vi "SDSU_REGS.vi"(0 "refnum":i32, 5 "Command":string, 7 "physical unit":string, 9 "swhitches":string[](array[string]), 11 "error in (no error)":errorcluster, 12 "switch arguments":string[](array[string])) -> (4 "refnum out":i32, 6 "response":string, 15 "error out":errorcluster)   [LabVIEW 2016]
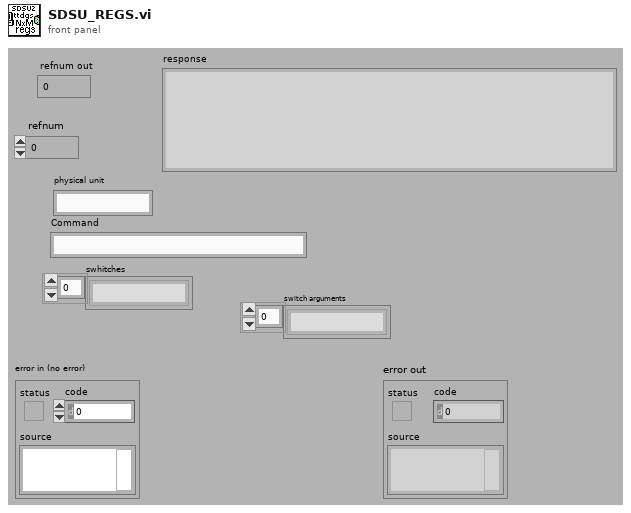
[diagram p1: front panel]
types:
  T1 = enum16{"READ FROM FILE", "GET ALL", "FIND BY NAME", "SET FIELD VALUE", "CLEAN"}
  T2 = typedef "CMN_ContStatus.ctl" = cluster{"Response":string, "power":bool, "shutter":bool, "artifdata":bool, "idlemode":bool, "reset":bool, "gain":u8, "speed":u8, "resetPCI":bool, "autoshutter":bool, "TempSetPoint":i32, "multipleextensions":bool, "displayImage":bool, "coadding":bool, "images being coadded":i32, "Operation Mode":enum16{"normal", "coadd", "fawler"}, "frames to write":cluster{"subs":bool, "reset":bool, "exposed":bool}, "fawler samples":i32, "write auto":bool, "datatype":string, "frames to display":cluster{"subs":bool, "reset":bool, "exposed":bool}, "sur":i32, "autoclear":bool}
  T3 = typedef "SDSU_Register.ctl" = cluster{"Name":string, "address":i16, "width":i16, "comment":string, "Fields":T4[], "value":string}
  T4 = typedef "SDSU_RegField.ctl" = cluster{"name":string, "position":u16, "num_bits":u16, "default":i16, "comment":string, "value":i32}
  T5 = enum16{"Idle", "Exposing", "Paused", "AbortExp", "Reading", "AbortRead", "FinishedReading", "Resetting", "Reducing", "Initializing"}
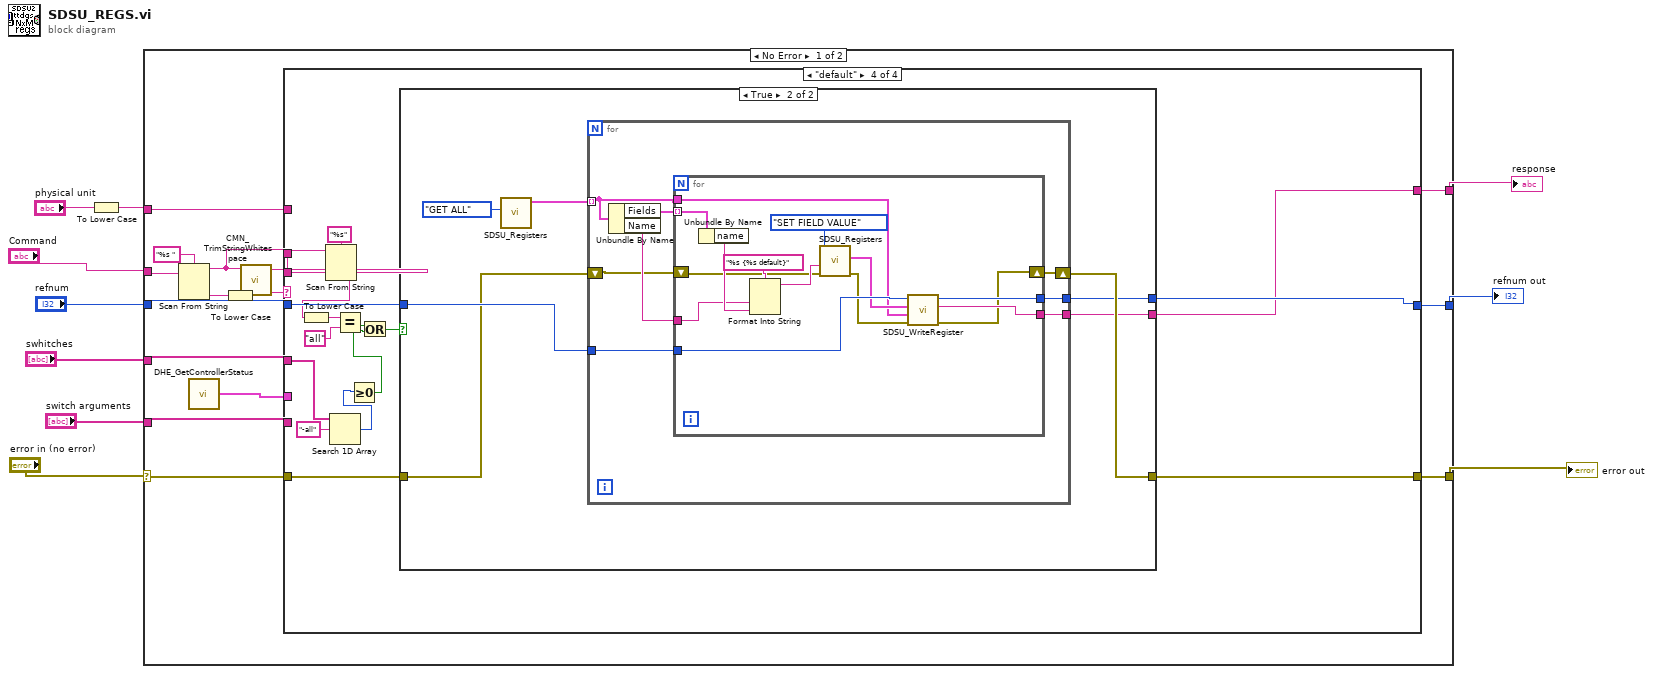
[diagram p0: block diagram]
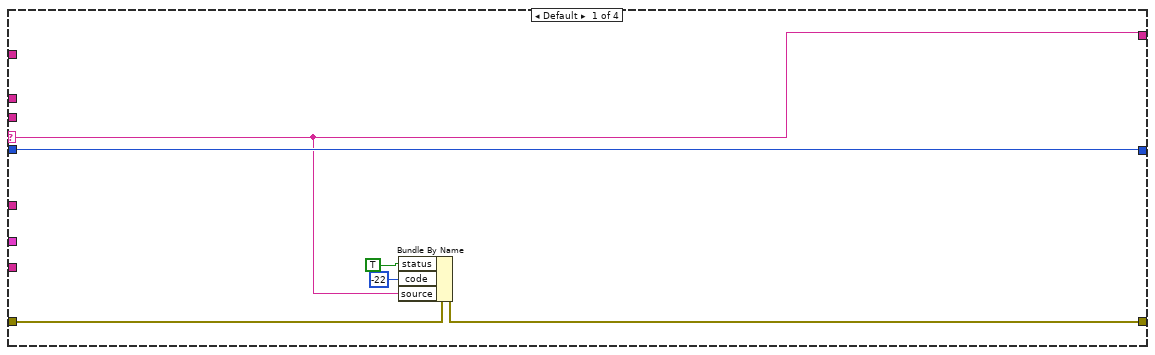
[diagram p2: hidden frame]
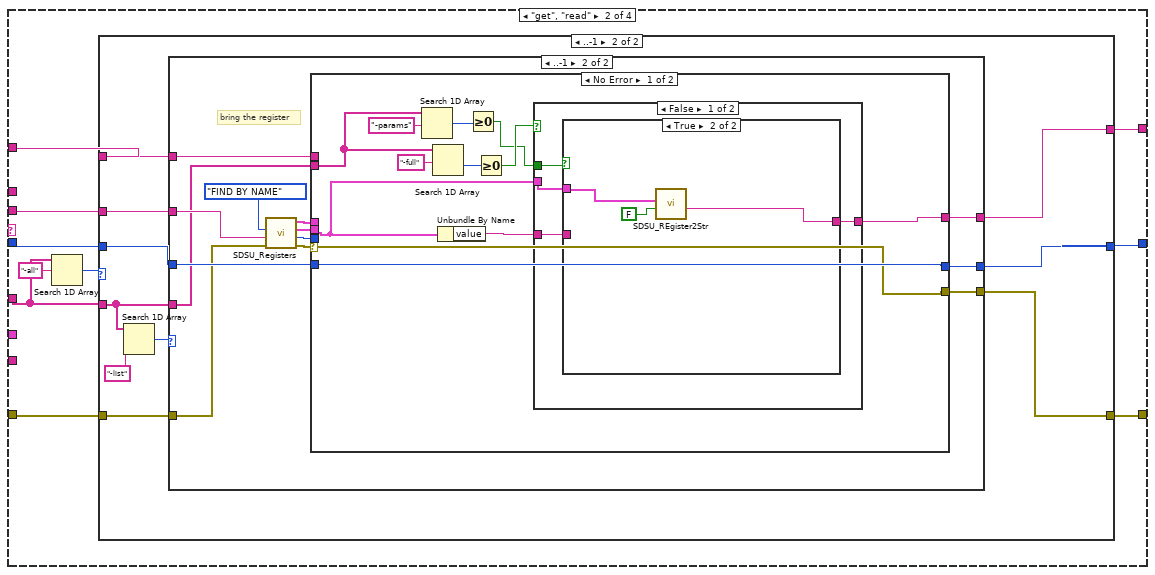
[diagram p3: hidden frame]
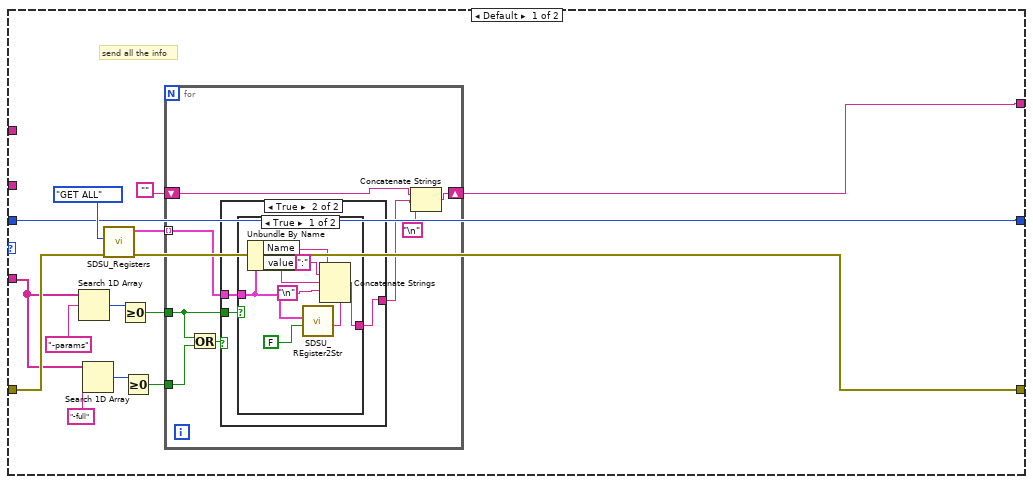
[diagram p4: hidden frame]
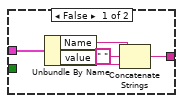
[diagram p5: hidden frame]
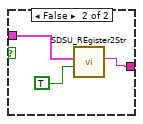
[diagram p6: hidden frame]
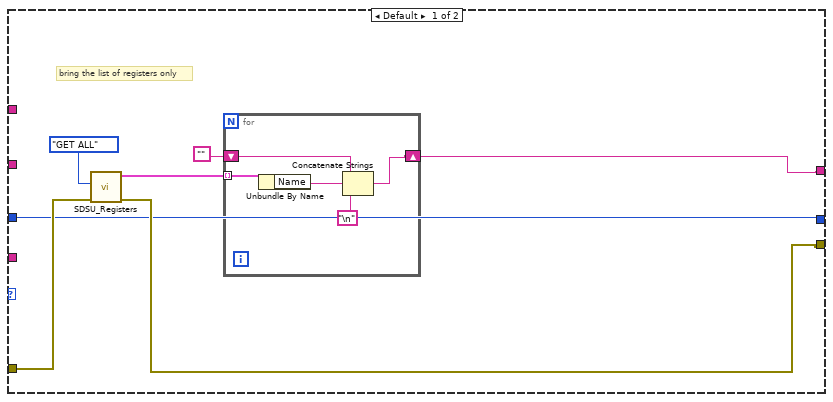
[diagram p7: hidden frame]
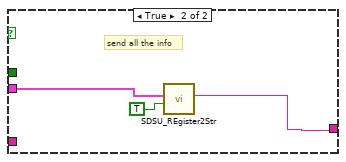
[diagram p9: hidden frame]
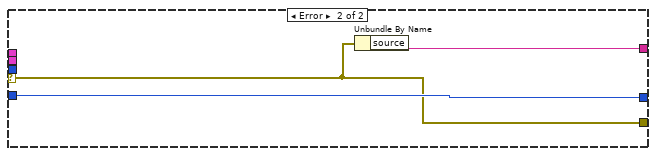
[diagram p10: hidden frame]
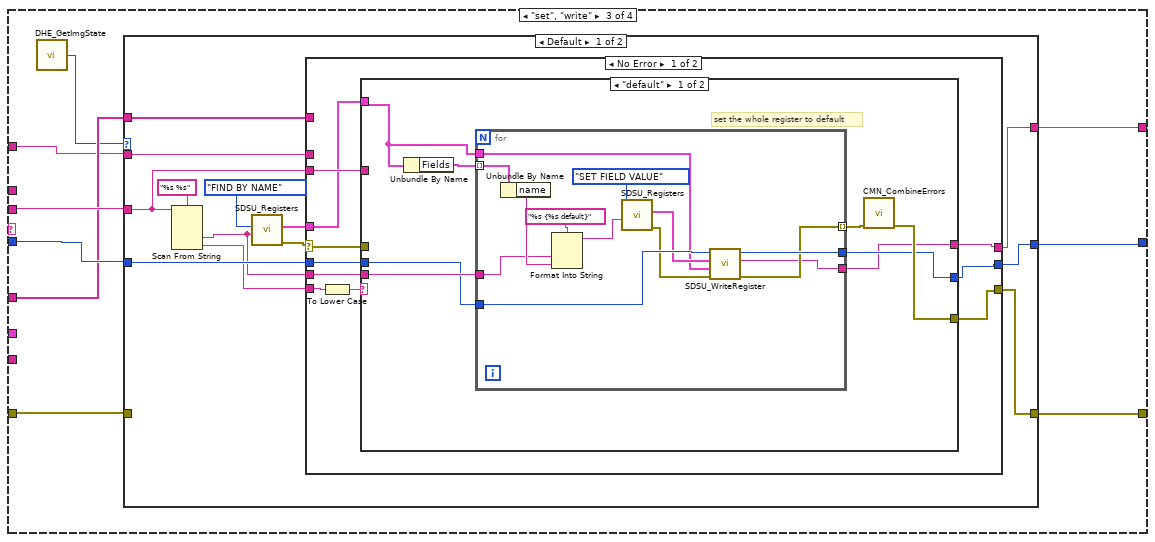
[diagram p11: hidden frame]
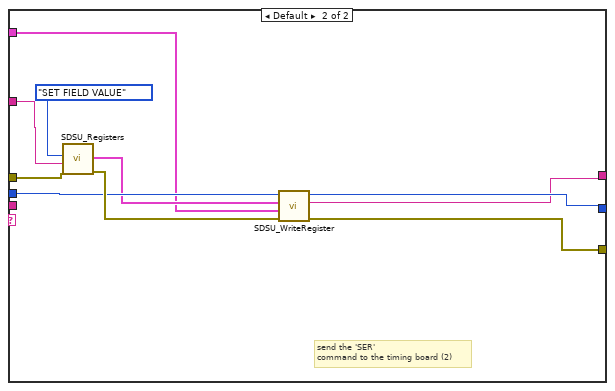
[diagram p12: hidden frame]
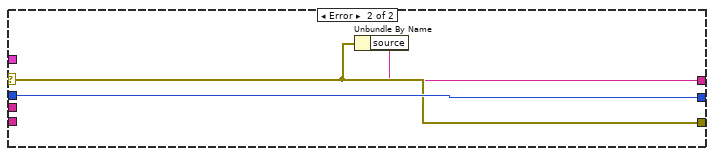
[diagram p13: hidden frame]
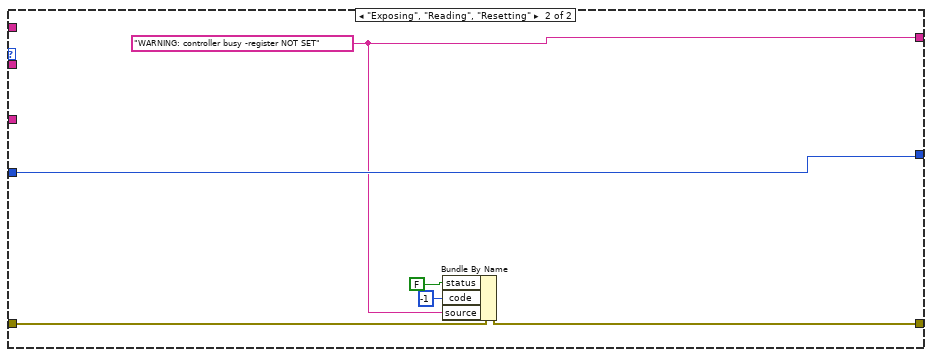
[diagram p14: hidden frame]
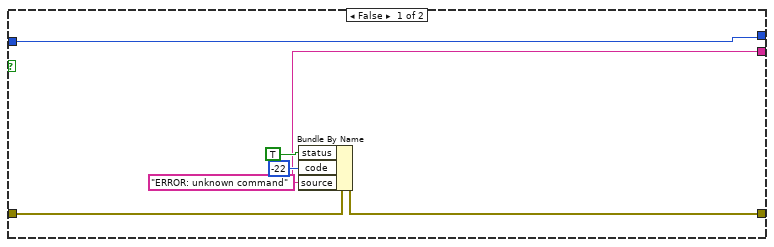
[diagram p15: hidden frame]
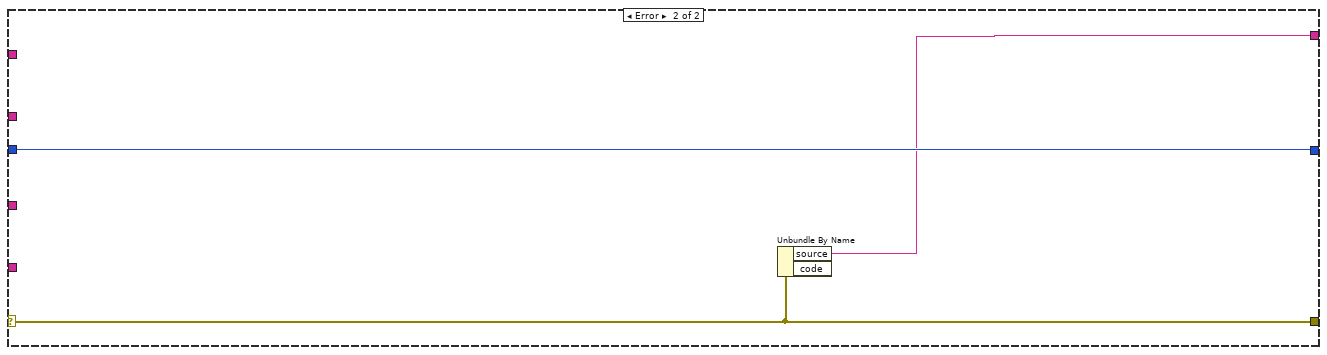
[diagram p16: hidden frame]
diagram:
  n1 = To Lower Case(string="physical unit") -> (all lower case string=w5:string)
  n2 = case shown="No Error" "error in (no error)" {
    selector: "error in (no error)" -> [w12 w267]
    tunnel: [w25 w267] -> w8
    tunnel: "refnum" -> [w24 w269]
    tunnel: [w23 w269] -> w10
    tunnel: "Command" -> [w16 _]
    tunnel: w5 -> [w15 _]
    tunnel: [w14 w268] -> w4
    tunnel: "swhitches" -> [w13 _]
    tunnel: "switch arguments" -> [w11 _]
    frame No Error {
      n3 = Scan From String(format string="%s " ("Format String"), input string=w16) -> (remaining string=w18:string, output 1=w19:string)  [unwired: 2 in, 3 out]
      n4 = call "DHE_GetControllerStatus.vi"() -> ("ControllerStatus"=w17:T2)  [unwired: 11 out]
      n5 = To Lower Case(string=w19) -> (all lower case string=w20:string)
      n6 = call "CMN_TrimStringWhitespace.vi"("string"=w18) -> ("trimmed string"=w21:string)  [unwired: 1 in, 8 out]
      n7 = case shown="\"default\"" w20 {
        selector: w20 -> [w26 _ _ _]
        tunnel: w12 -> [w31 w36 w151 w220]
        tunnel: [w30 w35 w149 w219] -> w25
        tunnel: w24 -> [w29 w37 w147 w231]
        tunnel: [w29 w41 w150 w218] -> w23
        tunnel: w21 -> [_ w38 w152 w226]
        tunnel: w17 -> [_ _ _ _]
        tunnel: w18 -> [_ _ _ _]
        tunnel: w15 -> [_ w39 w145 _]
        tunnel: [w26 w40 w148 w217] -> w14
        tunnel: w13 -> [_ w34 w146 w216]
        tunnel: w11 -> [_ _ _ _]
        frame Default {
          n8 = Bundle By Name(cluster=w31, "status"=TRUE, "code"=-22, "source"=w26) -> (w30:errorcluster)
        }
        frame "get", "read" {
          n9 = Search 1D Array(1D array=w34, element="-all") -> (index of element=w32:i32)  [unwired: 1 out]
          n10 = case shown="..-1" w32 {
            tunnel: [w44 w92] -> w41
            tunnel: [w45 w91] -> w40
            tunnel: w39 -> [_ w90]
            tunnel: w38 -> [_ w89]
            tunnel: w37 -> [w44 w88]
            tunnel: w34 -> [w50 w85]
            tunnel: w36 -> [w55 w87]
            tunnel: [w43 w86] -> w35
            frame Default {
              # "send all the info"
              n11 = Search 1D Array(1D array=w50, element="-params") -> (index of element=w48:i32)  [unwired: 1 out]
              n12 = Search 1D Array(1D array=w50, element="-full") -> (index of element=w49:i32)  [unwired: 1 out]
              n13 = call "SDSU_Registers.vi"("error in (no error)"=w55, "action"=T1."GET ALL") -> ("error out"=w43:errorcluster, "Registers"=w53:T3[])  [unwired: 2 in, 6 out]
              n14 = Greater Or Equal To 0?(x=w48) -> (x >= 0?=w47:bool)
              n15 = Greater Or Equal To 0?(x=w49) -> (x >= 0?=w46:bool)
              n16 = for {
                tunnel: w53 -> [w61] mode=indexing
                tunnel: w47 -> [w56]
                tunnel: w46 -> [w63]
                shift-right: [w60] -> w45
                shift-left: "" -> [w58]
                n17 = Or(x=w56, y=w63) -> (x .or. y?=w62:bool)
                n18 = case shown="True" w62 {
                  tunnel: w61 -> [w68 w70]
                  tunnel: [w64 w69] -> w59
                  tunnel: w56 -> [_ w71]
                  frame False {
                    n19 = Unbundle By Name(w68) -> ("Name"=w67:string, "value"=w66:string)
                    n20 = Concatenate Strings(w67, " " ("string"), w66) -> (w64:string)
                  }
                  frame True {
                    n21 = case shown="True" w71 {
                      tunnel: w70 -> [w78 w81]
                      tunnel: [w73 w80] -> w69
                      frame True {
                        n22 = Unbundle By Name(w78) -> ("Name"=w77:string, "value"=w72:string)
                        n23 = call "SDSU_REgister2Str.vi"("send comment"=FALSE, "Register"=w78) -> ("fields info"=w74:string)  [unwired: 9 out]
                        n24 = Concatenate Strings(w77, ":" ("string"), w72, "\n", w74) -> (w73:string)
                      }
                      frame False {
                        n25 = call "SDSU_REgister2Str.vi"("send comment"=TRUE, "Register"=w81) -> ("full info"=w80:string)  [unwired: 9 out]
                      }
                    }
                  }
                }
                n26 = Concatenate Strings(w58, w59, "\n") -> (w60:string)
              }
            }
            frame ..-1 {
              n27 = Search 1D Array(1D array=w85, element="-list") -> (index of element=w83:i32)  [unwired: 1 out]
              n28 = case shown="..-1" w83 {
                tunnel: [w94 w117] -> w92
                tunnel: [w96 w116] -> w91
                tunnel: w90 -> [_ w115]
                tunnel: w89 -> [_ w114]
                tunnel: w88 -> [w94 w113]
                tunnel: w85 -> [_ w112]
                tunnel: w87 -> [w98 w111]
                tunnel: [w95 w110] -> w86
                frame Default {
                  # "bring the list of registers only"
                  n29 = call "SDSU_Registers.vi"("error in (no error)"=w98, "action"=T1."GET ALL") -> ("error out"=w95:errorcluster, "Registers"=w97:T3[])  [unwired: 2 in, 6 out]
                  n30 = for {
                    tunnel: w97 -> [w104] mode=indexing
                    shift-right: [w102] -> w96
                    shift-left: "" -> [w101]
                    n31 = Unbundle By Name(w104) -> ("Name"=w103:string)
                    n32 = Concatenate Strings(w101, w103, "\n") -> (w102:string)
                  }
                }
                frame ..-1 {
                  # "bring the register"
                  n33 = call "SDSU_Registers.vi"("error in (no error)"=w111, "argument"=w114, "action"=T1."FIND BY NAME") -> ("error out"=w109:errorcluster, "index"=w107:i32, "Register"=w105:T3, "Registers"=w108:T3[])  [unwired: 1 in, 4 out]
                  n34 = case shown="No Error" w109 {
                    selector: w109 -> [w128 w142]
                    tunnel: w108 -> [_ _]
                    tunnel: w113 -> [w129 w143]
                    tunnel: [w129 w143] -> w117
                    tunnel: [w128 w142] -> w110
                    tunnel: [w125 w141] -> w116
                    tunnel: w115 -> [_ _]
                    tunnel: w107 -> [_ _]
                    tunnel: w112 -> [w121 _]
                    tunnel: w105 -> [w124 _]
                    frame No Error {
                      n35 = Search 1D Array(1D array=w121, element="-params") -> (index of element=w126:i32)  [unwired: 1 out]
                      n36 = Search 1D Array(1D array=w121, element="-full") -> (index of element=w120:i32)  [unwired: 1 out]
                      n37 = Unbundle By Name(w124) -> ("value"=w123:string)
                      n38 = Greater Or Equal To 0?(x=w126) -> (x >= 0?=w118:bool)
                      n39 = Greater Or Equal To 0?(x=w120) -> (x >= 0?=w119:bool)
                      n40 = case shown="False" w119 {
                        tunnel: [w131 w138] -> w125
                        tunnel: w124 -> [w133 w139]
                        tunnel: w123 -> [w130 _]
                        tunnel: w118 -> [w132 _]
                        frame False {
                          n41 = case shown="True" w132 {
                            tunnel: w133 -> [_ w136]
                            tunnel: [w134 w135] -> w131
                            tunnel: w130 -> [w134 _]
                            frame False {
                              # "value only"
                            }
                            frame True {
                              n42 = call "SDSU_REgister2Str.vi"("send comment"=FALSE, "Register"=w136) -> ("fields info"=w135:string)  [unwired: 9 out]
                            }
                          }
                        }
                        frame True {
                          # "send all the info"
                          n43 = call "SDSU_REgister2Str.vi"("send comment"=TRUE, "Register"=w139) -> ("full info"=w138:string)  [unwired: 9 out]
                        }
                      }
                    }
                    frame Error {
                      n44 = Unbundle By Name(w142) -> ("source"=w141:string)
                    }
                  }
                }
              }
            }
          }
        }
        frame "set", "write" {
          n45 = call "DHE_GetImgState.vi"() -> ("DHE_ImgState"=w144:T5)  [unwired: 9 out]
          n46 = case shown="Default" w144 {
            tunnel: w152 -> [w157 _]
            tunnel: w151 -> [_ w214]
            tunnel: [w165 w215] -> w150
            tunnel: [w164 w211] -> w149
            tunnel: [w163 w210] -> w148
            tunnel: w147 -> [w162 w215]
            tunnel: w146 -> [w161 _]
            tunnel: w145 -> [w160 _]
            frame Default {
              n47 = Scan From String(format string="%s %s", input string=w157) -> (output 1=w153:string, output 2=w154:string)  [unwired: 2 in, 5 out]
              n48 = call "SDSU_Registers.vi"("argument"=w153, "action"=T1."FIND BY NAME") -> ("error out"=w156:errorcluster, "Register"=w155:T3)  [unwired: 2 in, 6 out]
              n49 = case shown="No Error" w156 {
                selector: w156 -> [w174 w208]
                tunnel: w162 -> [w173 w209]
                tunnel: [w172 w209] -> w165
                tunnel: [w171 w208] -> w164
                tunnel: [w170 w207] -> w163
                tunnel: w161 -> [_ _]
                tunnel: w160 -> [_ _]
                tunnel: w157 -> [w175 _]
                tunnel: w155 -> [w169 _]
                tunnel: w154 -> [w168 _]
                tunnel: w153 -> [w166 _]
                frame No Error {
                  n50 = To Lower Case(string=w168) -> (all lower case string=w167:string)
                  n51 = case shown="\"default\"" w167 {
                    tunnel: w175 -> [_ w205]
                    tunnel: w174 -> [_ w204]
                    tunnel: w173 -> [w179 w202]
                    tunnel: [w178 w201] -> w172
                    tunnel: [w180 w197] -> w171
                    tunnel: [w176 w200] -> w170
                    tunnel: w169 -> [w177 w198]
                    tunnel: w166 -> [w182 _]
                    frame "default" {
                      # "set the whole register to default"
                      n52 = Unbundle By Name(w177) -> ("Fields"=w183:T4[])
                      n53 = for {
                        tunnel: w183 -> [w195] mode=indexing
                        tunnel: w182 -> [w192]
                        tunnel: [w187] -> w181 mode=indexing
                        tunnel: w179 -> [w190]
                        tunnel: [w189] -> w178
                        tunnel: w177 -> [w185]
                        tunnel: [w184] -> w176
                        n54 = Unbundle By Name(w195) -> ("name"=w193:string)
                        n55 = Format Into String(format string="%s {%s default}", w192, w193) -> (resulting string=w191:string)  [unwired: 2 in, 1 out]
                        n56 = call "SDSU_Registers.vi"("argument"=w191, "action"=T1."SET FIELD VALUE") -> ("error out"=w188:errorcluster, "Register"=w186:T3)  [unwired: 2 in, 6 out]
                        n57 = call "SDSU_WriteRegister.vi"("error in (no error)"=w188, "original Register"=w185, "new Register"=w186, "fd in"=w190) -> ("error out"=w187:errorcluster, "response"=w184:string, "fd out"=w189:i32)  [unwired: 5 out]
                      }
                      n58 = call "CMN_CombineErrors.vi"("Errors"=w181) -> ("error out"=w180:errorcluster)  [unwired: 10 out]
                    }
                    frame Default {
                      # "send the 'SER'\ncommand to the timing board (2)"
                      n59 = call "SDSU_Registers.vi"("error in (no error)"=w204, "argument"=w205, "action"=T1."SET FIELD VALUE") -> ("error out"=w203:errorcluster, "Register"=w199:T3)  [unwired: 1 in, 6 out]
                      n60 = call "SDSU_WriteRegister.vi"("error in (no error)"=w203, "original Register"=w198, "new Register"=w199, "fd in"=w202) -> ("error out"=w197:errorcluster, "response"=w200:string, "fd out"=w201:i32)  [unwired: 5 out]
                    }
                  }
                }
                frame Error {
                  n61 = Unbundle By Name(w208) -> ("source"=w207:string)
                }
              }
            }
            frame "Exposing", "Reading", "Resetting" {
              w210 = "WARNING: controller busy -register NOT SET" ("source")
              n62 = Bundle By Name(cluster=w214, "status"=FALSE, "code"=-1, "source"=w210) -> (w211:errorcluster)
            }
          }
        }
        frame "default" {
          n63 = Scan From String(format string="%s", input string=w226) -> (output 1=w223:string)  [unwired: 2 in, 4 out]
          n64 = To Lower Case(string=w223) -> (all lower case string=w222:string)
          n65 = Search 1D Array(1D array=w216, element="-all") -> (index of element=w229:i32)  [unwired: 1 out]
          n66 = Equal?(x=w222, y="all") -> (x = y?=w224:bool)
          n67 = Greater Or Equal To 0?(x=w229) -> (x >= 0?=w228:bool)
          n68 = Or(x=w224, y=w228) -> (x .or. y?=w227:bool)
          n69 = case shown="True" w227 {
            tunnel: w231 -> [w233 w242]
            tunnel: w220 -> [w237 w241]
            tunnel: [w236 w240] -> w219
            tunnel: [w233 w239] -> w218
            tunnel: [w232 w238] -> w217
            frame False {
              w232 = "ERROR: unknown command" ("source")
              n70 = Bundle By Name(cluster=w237, "status"=TRUE, "code"=-22, "source"=w232) -> (w236:errorcluster)
            }
            frame True {
              n71 = call "SDSU_Registers.vi"("action"=T1."GET ALL") -> ("Registers"=w243:T3[])  [unwired: 3 in, 7 out]
              n72 = for {
                tunnel: w243 -> [w251] mode=indexing
                tunnel: w242 -> [w249]
                tunnel: [w248] -> w239
                shift-right: [w247] -> w240
                shift-left: w241 -> [w246]
                tunnel: [w245] -> w238
                n73 = Unbundle By Name(w251) -> ("Fields"=w252:T4[], "Name"=w250:string)
                n74 = for {
                  tunnel: w252 -> [w265] mode=indexing
                  tunnel: w250 -> [w262]
                  tunnel: w249 -> [w260]
                  tunnel: [w259] -> w248
                  tunnel: w251 -> [w256]
                  tunnel: [w255] -> w245
                  shift-right: [w254] -> w247
                  shift-left: w246 -> [w253]
                  n75 = Unbundle By Name(w265) -> ("name"=w263:string)
                  n76 = Format Into String(format string="%s {%s default}", w262, w263) -> (resulting string=w261:string)  [unwired: 2 in, 1 out]
                  n77 = call "SDSU_Registers.vi"("error in (no error)"=w253, "argument"=w261, "action"=T1."SET FIELD VALUE") -> ("error out"=w258:errorcluster, "Register"=w257:T3)  [unwired: 1 in, 6 out]
                  n78 = call "SDSU_WriteRegister.vi"("error in (no error)"=w258, "original Register"=w256, "new Register"=w257, "fd in"=w260) -> ("error out"=w254:errorcluster, "response"=w255:string, "fd out"=w259:i32)  [unwired: 5 out]
                }
              }
            }
          }
        }
      }
    }
    frame Error {
      n79 = Unbundle By Name(w267) -> ("source"=w268:string)  [unwired: 1 out]
    }
  }
  "refnum out" <- w10
  "error out" <- w8
  "response" <- w4
